vi "C-F_viawhile.vi"() -> ()   [LabVIEW 2024]
panel:
  out "no of i":i32
  in  "Boolean":bool
  out "F":dbl(slide) scale=0.0..300.0
  in  "c":dbl(slide) scale=0.0..100.0
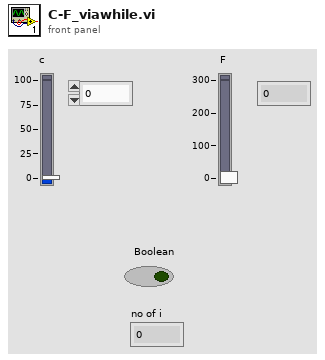
[diagram p1: front panel]
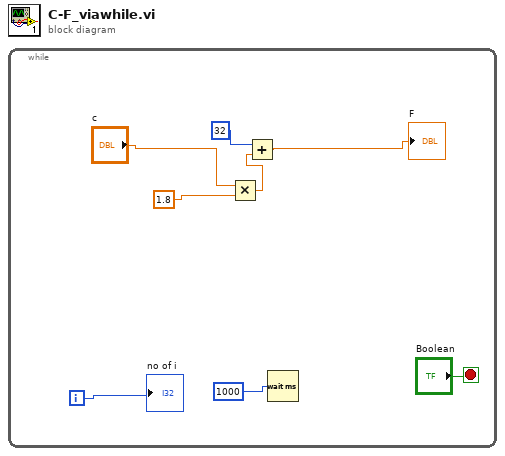
[diagram p0: block diagram]
diagram:
  n1 = while {
    i -> [w7]
    stop <- "Boolean" stop-if-true
    n2 = Multiply(x="c", y=1.8) -> (x*y=w3:dbl)
    n3 = Add(x=32, y=w3) -> (x+y=→"F":dbl)
    n4 = Wait (ms)(milliseconds to wait=u32 1000 ("millisecond timer value")) -> ()  [unwired: 1 out]
    "no of i" <- w7
  }
